vi "AC2250 Initialize.vi"(8 "ErrIn":errorcluster, 11 "VISA Resource Name In":refnum<visa-resource-name>) -> (0 "ErrOut":errorcluster, 3 "VISA Resource Name Out":refnum<visa-resource-name>)   [LabVIEW 2013]
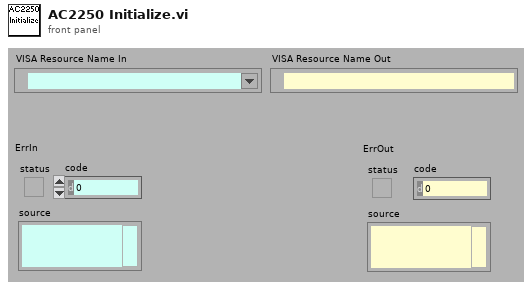
[diagram p1: front panel]
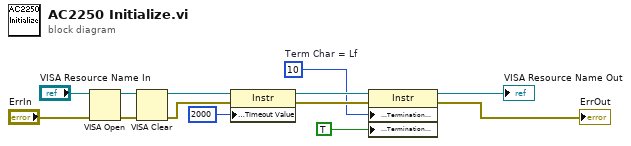
[diagram p0: block diagram]
diagram:
  w2 = u8 10  # Term Char = Lf
  n1 = VISA Open(error in (no error)="ErrIn", VISA resource name="VISA Resource Name In") -> (VISA resource name=w11:refnum<visa-resource-name>, error out=w10:errorcluster)  [unwired: 3 in]
  n2 = VISA Clear(VISA resource name=w11, error in (no error)=w10) -> (VISA resource name out=w8:refnum<visa-resource-name>, error out=w7:errorcluster)
  n3 = property class="Instr"(reference=w8, error in=w7, "General Settings:Timeout Value"=u32 2000) -> (reference out=w6:refnum<visa-resource-name>, error out=w5:errorcluster)
  n4 = property class="Instr"(reference=w6, error in=w5, "Message Based Settings:Termination Character"=w2, "Message Based Settings:Termination Character Enable"=TRUE) -> (reference out=→"VISA Resource Name Out":refnum<visa-resource-name>, error out=→"ErrOut":errorcluster)
